vi "Set Acceleration.vi"(6 "Units (0: data)":u16(ring) items=["device units", "microns/s^2", "mm/s^2", "inches/s^2", "degrees/s^2"], 7 "New Acceleration":dbl, 8 "error in (no error)":errorcluster, 9 "Device and Axis":string, 10 "Microstep Size (0)":dbl, 11 "VISA resource name":refnum<visa-resource-name>) -> (0 "error out":errorcluster, 3 "VISA resource name out":refnum<visa-resource-name>)   [LabVIEW 2018, in "Zaber A Series.lvlib"]
doc: "Sets the acceleration and deceleration of a device to a new value. The desired acceleration and units of measure are inputs. If the acceleration input is zero, then it won't be updated. The units for the acceleration can be selected with the Units input. 'Data' units are the default, and other unit selections require the Microstep Size for the device to be input. If you'd like to specify a Device and Axis to adjust the settings of, specify this input.\n\nThis VI requires that the Initialize VI has been called with the same serial port."
uses:
  Zaber A Series.lvlib
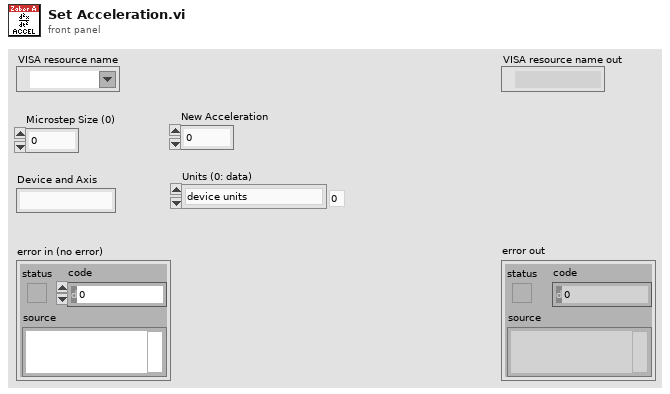
[diagram p1: front panel]
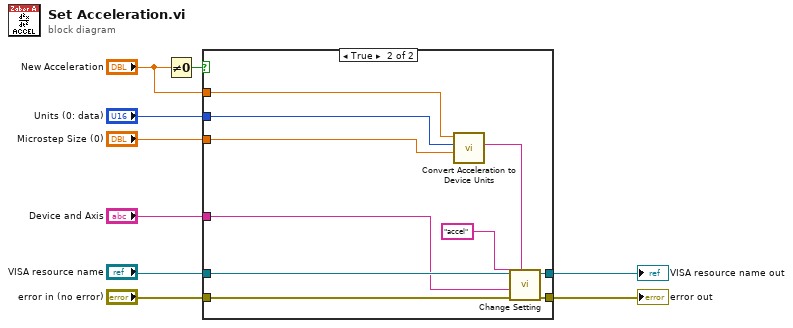
[diagram p0: block diagram]
diagram:
  n1 = Not Equal To 0?(x="New Acceleration") -> (x != 0?=w9:bool)
  n2 = case shown="True" w9 {
    tunnel: "VISA resource name" -> [w11 w17]
    tunnel: [w11 w21] -> w7
    tunnel: "error in (no error)" -> [w10 w19]
    tunnel: [w10 w20] -> w6
    tunnel: "Microstep Size (0)" -> [_ w13]
    tunnel: "Units (0: data)" -> [_ w14]
    tunnel: "Device and Axis" -> [_ w16]
    tunnel: "New Acceleration" -> [_ w15]
    frame False {
    }
    frame True {
      n3 = call "Convert Acceleration to Device Units.vi"("Microstep Size (0)"=w13, "Units (0: device acceleration units)"=w14, "Acceleration (0)"=w15) -> ("Device Acceleration (String)"=w12:string)  [unwired: 6 in, 2 out]
      n4 = call "Change Setting.vi"("Data"=w12, "error in (no error)"=w19, "Device and Axis"=w16, "Setting"="accel" ("Common Settings"), "VISA resource name"=w17) -> ("error out"=w20:errorcluster, "VISA resource name out"=w21:refnum<visa-resource-name>)  [unwired: 5 in]
    }
  }
  "VISA resource name out" <- w7
  "error out" <- w6
